vi "Write Stamina.vi"(8 "error in (no error)":errorcluster, 10 "Stamina":i32, 11 "Peasant in":refnum<class "Peasant.lvclass">) -> (0 "error out":errorcluster, 3 "Peasant out":refnum<class "Peasant.lvclass">)   [LabVIEW 2021]
uses:
  Peasant.lvclass
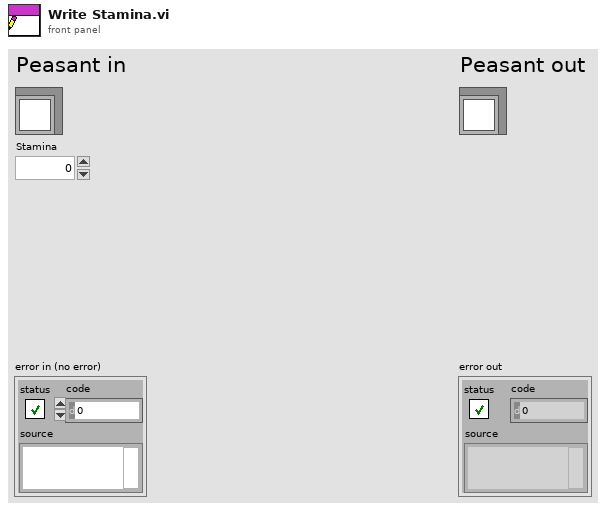
[diagram p1: front panel]
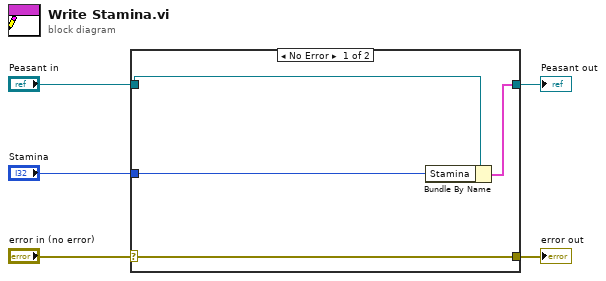
[diagram p0: block diagram]
diagram:
  n1 = case shown="No Error" "error in (no error)" {
    selector: "error in (no error)" -> [w9 w10]
    tunnel: [w9 w10] -> w4
    tunnel: [w7 w11] -> w2
    tunnel: "Peasant in" -> [w8 w11]
    tunnel: "Stamina" -> [w6 _]
    frame No Error {
      n2 = Bundle By Name(cluster=w8, "Stamina"=w6) -> (w7:cluster{})
    }
    frame Error {
    }
  }
  "error out" <- w4
  "Peasant out" <- w2
